vi "Initialize-status-notifs.vi"(8 "error in (no error)":errorcluster, 11 "Object ref in":T1) -> (0 "error out":errorcluster, 3 "Object ref out":T1)   [LabVIEW 2013, in "HardwareCharacterization.lvlib" / "HC-Main.lvclass"]
uses:
  HC-Main.lvclass
  Object-reference.ctl
  HC-Main.lvclass/HC-Main.ctl
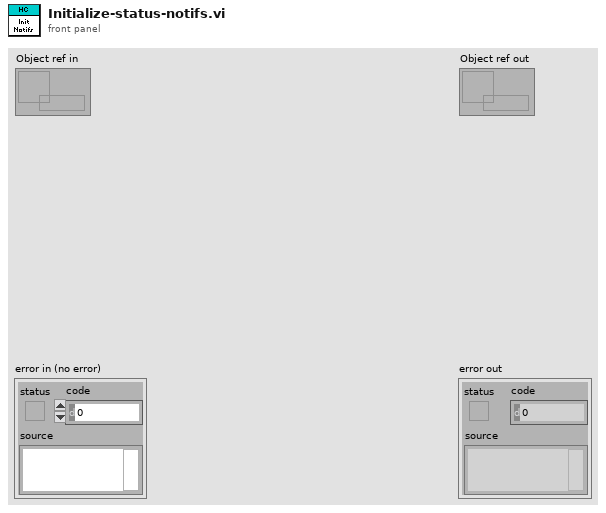
[diagram p1: front panel]
types:
  T1 = typedef "HardwareCharacterization.lvlib/HC-Main.lvclass/Object-reference.ctl" = refnum<data-value>
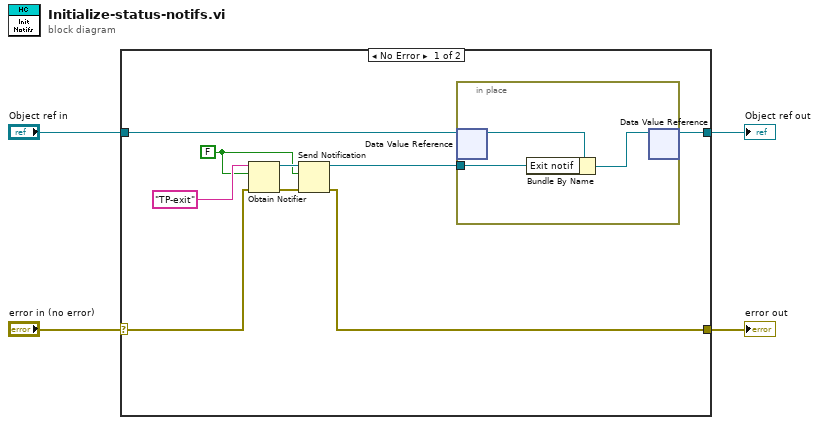
[diagram p0: block diagram]
diagram:
  n1 = case shown="No Error" "error in (no error)" {
    selector: "error in (no error)" -> [w5 w18]
    tunnel: [w6 w18] -> w3
    tunnel: [w12 w17] -> w1
    tunnel: "Object ref in" -> [w13 w17]
    frame No Error {
      w7 = FALSE
      n2 = Obtain Notifier(name (unnamed)="TP-exit", notification data type=w7, error in (no error)=w5) -> (notifier out=w11:refnum<notifier>, error out=w8:errorcluster)  [unwired: 1 in, 1 out]
      n3 = Send Notification(notification=w7, notifier=w11, error in (no error)=w8) -> (notifier out=w9:refnum<notifier>, error out=w6:errorcluster)
      n4 = in-place {
        in-place-border: w9 -> [w14]
        n5 = in-place-dvr #1(w13) -> (w16:refnum<class "HC-Main.lvclass">)  [unwired: 1 out]
        n6 = Bundle By Name(cluster=w16, "Exit notif"=w14) -> (w15:refnum<class "HC-Main.lvclass">)
        n7 = in-place-dvr #1(w15) -> (w12:T1)  [unwired: 1 out]
      }
    }
    frame Error {
    }
  }
  "error out" <- w3
  "Object ref out" <- w1
